vi "MAIN_merFISH_start_autofocus.vi"(5 "queue FPGA":refnum<queue>, 6 "PID gains":T3={"proportional gain (Kc)"=50.0, "integral time (Ti, min)"=0.03, "derivative time (Td, min)"=0.0} {"derivative time (Td, min)" format="%.3f"; "integral time (Ti, min)" format="%.3f"; "proportional gain (Kc)" format="%.3f"}, 7 "queue piezo":refnum<queue>, 8 "error in":errorcluster, 9 "Starting time":dbl, 10 "Log file":refnum<file>, 11 "QPD ref":T1) -> (0 "error out":errorcluster, 3 "Next task":T2)   [LabVIEW 2015]
uses:
  CONTROLS/Q_main_element.ctl
  CONTROLS/Q_MCL_piezo_element.ctl
  CONTROLS/Q_FPGA_element.ctl
  GLOBAL/Global_MCL_piezo.vi
  GLOBAL/Global_ABORT.vi
panel:
  out "Stabilization":dbl
  out "Piezo":dbl
  out "FPGA":dbl
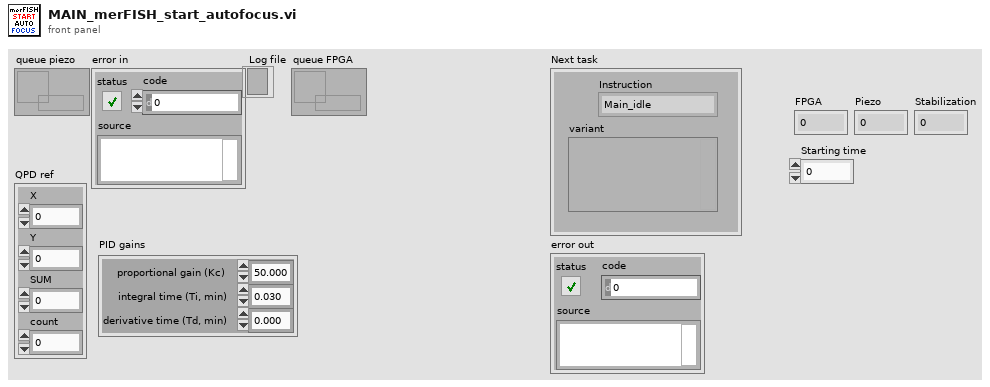
[diagram p1: front panel]
types:
  T1 = cluster{"X":sgl, "Y":sgl, "SUM":sgl, "count":u32}
  T2 = typedef "Q_main_element.ctl" = cluster{"variant":variant, "Instruction":enum16{"Main_idle", "Main_initialize", "Main_initialize_TDMS", "Main_initialize_Queue", "Main_error", "Main_DAQ_initialization_results", "Main_ASI_initialization_results", "Main_Piezo_initialization_results", "Main_Valve_initialization_results", "Main_Pump_initialization_results", "Main_CAMERA_initialization_results", "Main_FPGA_initialization_results", "Main_DAQ_error", "Main_ASI_error", "Main_Piezo_error", "Main_CAMERA_error", "Main_Valve_error", "Main_Pump_error", "Main_FPGA_error", "Main_start_acquiring", "Main_not_acquiring", "Main_acquiring", "Main_stop_acquiring", "Main_change_exposure", "Main_change_z_scan_parameters", "Main_define_ROI", "Main_define_mosaic", "Main_read_kinetic_time", "Main_cooler", "Main_read_temperature", "Main_save_XY", "Main_load_XY", "Main_discard_XY", "Main_move_to_XY", "Main_measure_QPD", "Main_autofocus_calibration", "Main_autofocus_initialization", "Main_autofocus_stop", "Main_save_PID", "Main_change_H_valve_position", "Main_two_way_valve", "Main_save_movie", "Main_init_single_scan", "Main_single_scan", "Main_stop_single_scan", "Main_merFISH_illumination_parameters", "Main_merFISH_buffer_probe_list", "Main_merFISH_injections_procedure", "Main_merFISH_save_setpoint", "Main_merFISH_DAPI_parameters", "Main_merFISH_Brightfield_parameters", "Main_merFISH_save_embryo_ROI", "Main_merFISH_init", "Main_merFISH_resume", "Main_merFISH_start_autofocus", "Main_merFISH_open_close_valve_merFISH", "Main_merFISH_open_close_valve_photobleaching", "Main_merFISH_hybridization", "Main_merFISH_move_to_ROI", "Main_merFISH_wait_stabilization", "Main_merFISH_move_to_REF", "Main_merFISH_scan", "Main_merFISH_photobleaching_injection", "Main_merFISH_photobleaching", "Main_merFISH_send_email", "Main_merFISH_close", "Main_STOP"}}
  T3 = cluster{"proportional gain (Kc)":dbl, "integral time (Ti, min)":dbl, "derivative time (Td, min)":dbl}
  T4 = typedef "Q_FPGA_element.ctl" = cluster{"variant":variant, "Instruction":enum16{"FPGA_idle", "FPGA_initialize", "FPGA_error", "FPGA_security_stop", "FPGA_laser", "FPGA_start_stop_measure_QPD", "FPGA_measure_QPD", "FPGA_measure_QPD_noise", "FPGA_stop_measure_QPD", "FPGA_init_autofocus", "FPGA_init_single_scan", "FPGA_stop_single_scan", "FPGA_init_merFISH", "FPGA_measure_QPD_merFISH", "FPGA_init_scan_merFISH", "FPGA_scan_merFISH", "FPGA_close_merFISH", "FPGA_stop"}}
  T5 = typedef "Q_MCL_piezo_element.ctl" = cluster{"variant":variant, "Instruction":enum16{"Piezo_idle", "Piezo_initialize", "Piezo_error", "Piezo_security_stop", "Piezo_read_z", "Piezo_move_z", "Piezo_keyboard_move", "Piezo_close_autofocus_calibration_ramp", "Piezo_change_init_state", "Piezo_init_autofocus", "Piezo_init_autofocus_merFISH_TL", "Piezo_autofocus", "Piezo_autofocus_merFISH_TL", "Piezo_stop_autofocus", "Piezo_stop_autofocus_merFISH_TL", "Piezo_autofocus_lost", "Piezo_resume_autofocus_merFISH_TL", "Piezo_check_z_position_merFISH_TL", "Piezo_init_ramp", "Piezo_move_z_ramp", "Piezo_close_ramp", "Piezo_close_merFISH", "Piezo_stop"}}
  T6 = cluster{"PID gains":cluster{"proportional gain (Kc)":dbl, "integral time (Ti, min)":dbl, "derivative time (Td, min)":dbl}, "QPD ref":cluster{"X":sgl, "Y":sgl, "SUM":sgl, "count":u32}}
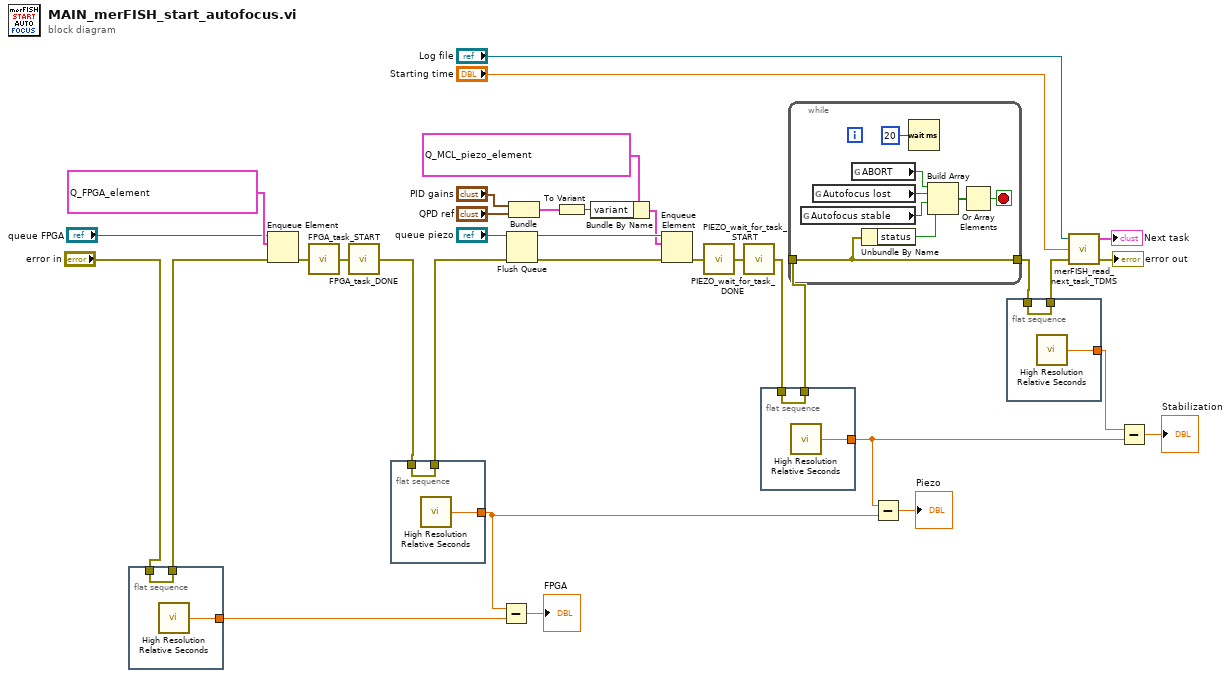
[diagram p0: block diagram]
diagram:
  n1 = flat-sequence {
    tunnel: "error in" -> [w36]
    tunnel: [w36] -> w14
    tunnel: [w35] -> w11
    frame #0 {
      n2 = call <vilib>:"High Resolution Relative Seconds.vi"() -> ("relative seconds"=w35:dbl)
    }
  }
  n3 = Enqueue Element(queue="queue FPGA", element=T4 {"variant"=variant, "Instruction"=enum."FPGA_measure_QPD_merFISH"}, error in (no error)=w14) -> (error out=w18:errorcluster)  [unwired: 1 in, 2 out]
  n4 = call "FPGA_task_START.vi"("error in"=w18) -> ("error out"=w19:errorcluster)
  n5 = call "FPGA_task_DONE.vi"("error in"=w19) -> ("error out"=w13:errorcluster)
  n6 = flat-sequence {
    tunnel: w13 -> [w38]
    tunnel: [w38] -> w12
    tunnel: [w37] -> w6
    frame #0 {
      n7 = call <vilib>:"High Resolution Relative Seconds.vi"() -> ("relative seconds"=w37:dbl)
    }
  }
  n8 = Subtract(x=w6, y=w11) -> (x-y=→"FPGA":dbl)
  n9 = Flush Queue(queue="queue piezo", error in (no error)=w12) -> (queue out=w31:refnum<queue>, error out=w32:errorcluster)  [unwired: 1 out]
  n10 = Bundle("PID gains"="PID gains", "QPD ref"="QPD ref") -> (w28:T6)  [unwired: 1 in]
  n11 = To Variant(anything=w28) -> (Variant=w29:variant)
  n12 = Bundle By Name(cluster=T5 {"variant"=variant, "Instruction"=enum."Piezo_init_autofocus_merFISH_TL"} ("element"), "variant"=w29) -> (w27:T5)
  n13 = Enqueue Element(queue=w31, element=w27, error in (no error)=w32) -> (error out=w33:errorcluster)  [unwired: 1 in, 2 out]
  n14 = call "PIEZO_wait_for_task_START.vi"("error in"=w33) -> ("error out"=w34:errorcluster)
  n15 = call "PIEZO_wait_for_task_DONE.vi"("error in"=w34) -> ("error out"=w9:errorcluster)
  n16 = flat-sequence {
    tunnel: w9 -> [w40]
    tunnel: [w40] -> w8
    tunnel: [w39] -> w2
    frame #0 {
      n17 = call <vilib>:"High Resolution Relative Seconds.vi"() -> ("relative seconds"=w39:dbl)
    }
  }
  n18 = while {
    tunnel: [w42] -> w5
    tunnel: w8 -> [w42]
    stop <- w43 stop-if-true
    n19 = global read "Global_MCL_piezo.vi" "Autofocus stable"() -> (w45:bool)
    n20 = global read "Global_MCL_piezo.vi" "Autofocus lost"() -> (w47:bool)
    n21 = global read "Global_ABORT.vi" "ABORT"() -> (w46:bool)
    n22 = Unbundle By Name(w42) -> ("status"=w41:bool)
    n23 = Wait (ms)(milliseconds to wait=u32 20) -> ()  [unwired: 1 out]
    n24 = Build Array(w46, w47, w45, w41) -> (w44:bool[])
    n25 = Or Array Elements(Boolean array=w44) -> (logical OR=w43:bool)
  }
  n26 = Subtract(x=w2, y=w6) -> (x-y=→"Piezo":dbl)
  n27 = flat-sequence {
    tunnel: w5 -> [w50]
    tunnel: [w50] -> w4
    tunnel: [w49] -> w1
    frame #0 {
      n28 = call <vilib>:"High Resolution Relative Seconds.vi"() -> ("relative seconds"=w49:dbl)
    }
  }
  n29 = call "merFISH_read_next_task_TDMS.vi"("error in"=w4, "Starting time"="Starting time", "Log file"="Log file") -> ("error out"=→"error out":errorcluster, "task"=→"Next task":T2)  [unwired: 1 in]
  n30 = Subtract(x=w1, y=w2) -> (x-y=→"Stabilization":dbl)
